vi "FT10_Fornax Send MonopolarCommand.vi"(8 "error in":errorcluster, 10 "Set Monopolar Command Cluster in":T12={"Serial Number"="CAMM_INTERNAL_GENERIC", "EnergyChannelID"=enum."EC_MONO_1", "CutMode"=enum."SPRAY_MODE", "CoagMode"=enum."SPRAY_MODE", "CutPowerCommand"=enum."POWER_NO_CHANGE", "CoagPowerCommand"=enum."POWER_NO_CHANGE", "Fornax Set Monopolar Command"=FALSE}, 11 "Message Handling Cluster in":T1={"Fornax Connected?"=refnum, "Unitherm Connected?"=refnum, "M4X Connected?"=refnum, "Unitherm Connect/Disconnect"=refnum, "Fornax Connection"=refnum, "UNITHERM Connection"="", "M4X Connection"=0, "PXI-7854R FPGA Reference"=refnum, "PXI-7854R Connected?"=refnum, "Fornax Connect/Disconnect"=refnum, "7854 Connect/Disconnect"=refnum, "M4X Connect/Disconnect"=refnum, "Config Cluster"={"Unitherm Port"="COM4", "Simulate Values"=TRUE}, "Log Queue"=refnum, "Log Analysis Cluster"={"RMS"=0.0, "Envelope Frequency"=0.0, "Peak"=0.0, "Crest Factor"=0.0, "Duty Cyle %"=0.0, "P-P"=0.0, "Frequency"=0.0, "THD"=0.0, "Postive Peak"=0.0, "Negative Peak"=0.0, "Mag_H1"=0.0, "Phase_H1"=0.0, "Mag_H3"=0.0, "Phase_H3"=0.0, "Mag_H5"=0.0, "Phase_H5"=0.0}, "Log Waveform Cluster"={"t0"=timestamp(0 s since 1904-01-01), "dt"=1.0, "Y"=[]}, "Log Time"=timestamp(0 s since 1904-01-01), "Log Flag"=FALSE}) -> (0 "error out":errorcluster, 2 "Set Monopolar Command Cluster out":T12={"Serial Number"="CAMM_INTERNAL_GENERIC", "EnergyChannelID"=enum."EC_MONO_1", "CutMode"=enum."SPRAY_MODE", "CoagMode"=enum."SPRAY_MODE", "CutPowerCommand"=enum."POWER_NO_CHANGE", "CoagPowerCommand"=enum."POWER_NO_CHANGE", "Fornax Set Monopolar Command"=FALSE}, 3 "Message Handling Cluster out":T1={"Fornax Connected?"=refnum, "Unitherm Connected?"=refnum, "M4X Connected?"=refnum, "Unitherm Connect/Disconnect"=refnum, "Fornax Connection"=refnum, "UNITHERM Connection"="", "M4X Connection"=0, "PXI-7854R FPGA Reference"=refnum, "PXI-7854R Connected?"=refnum, "Fornax Connect/Disconnect"=refnum, "7854 Connect/Disconnect"=refnum, "M4X Connect/Disconnect"=refnum, "Config Cluster"={"Unitherm Port"="COM4", "Simulate Values"=TRUE}, "Log Queue"=refnum, "Log Analysis Cluster"={"RMS"=0.0, "Envelope Frequency"=0.0, "Peak"=0.0, "Crest Factor"=0.0, "Duty Cyle %"=0.0, "P-P"=0.0, "Frequency"=0.0, "THD"=0.0, "Postive Peak"=0.0, "Negative Peak"=0.0, "Mag_H1"=0.0, "Phase_H1"=0.0, "Mag_H3"=0.0, "Phase_H3"=0.0, "Mag_H5"=0.0, "Phase_H5"=0.0}, "Log Waveform Cluster"={"t0"=timestamp(0 s since 1904-01-01), "dt"=1.0, "Y"=[]}, "Log Time"=timestamp(0 s since 1904-01-01), "Log Flag"=FALSE})   [LabVIEW 2015]
uses:
  Controls/Control_Fornax Set Monopolar Command Cluster.ctl
  Controls/Control_Fornax Set Monopolar Command - Serial Number String.ctl
  Controls/Control_Fornax Set Monopolar Command - Energy Channel ID Enum.ctl
  Controls/Control_Fornax Set Monopolar Command - Cut Mode Enum.ctl
  Controls/Control_Fornax Set Monopolar Command - Coag Mode Enum.ctl
  Controls/Control_Fornax Set Monopolar Command - Cut Power Command Enum.ctl
  Controls/Control_Fornax Set Monopolar Command - Coag Power Command Enum.ctl
  Controls/Control_Fornax Set Monopolar Command Bool.ctl
  Controls/Control_Message Handling Cluster.ctl
  Controls/Control_M4X Connection.ctl
  Controls/Control_PXI-7854R FPGA Reference.ctl
  Controls/Control_Config Cluster.ctl
  Controls/Control_Config Unitherm Port.ctl
  Controls/Control_Config Simulate Values.ctl
  Controls/Control_Log Queue.ctl
  Controls/Control_Log Cluster.ctl
  Controls/Control_Log Time.ctl
  Controls/Control_Log Waveform Cluster.ctl
  Controls/Control_Log Analysis Cluster.ctl
  Controls/Control_Log Flag.ctl
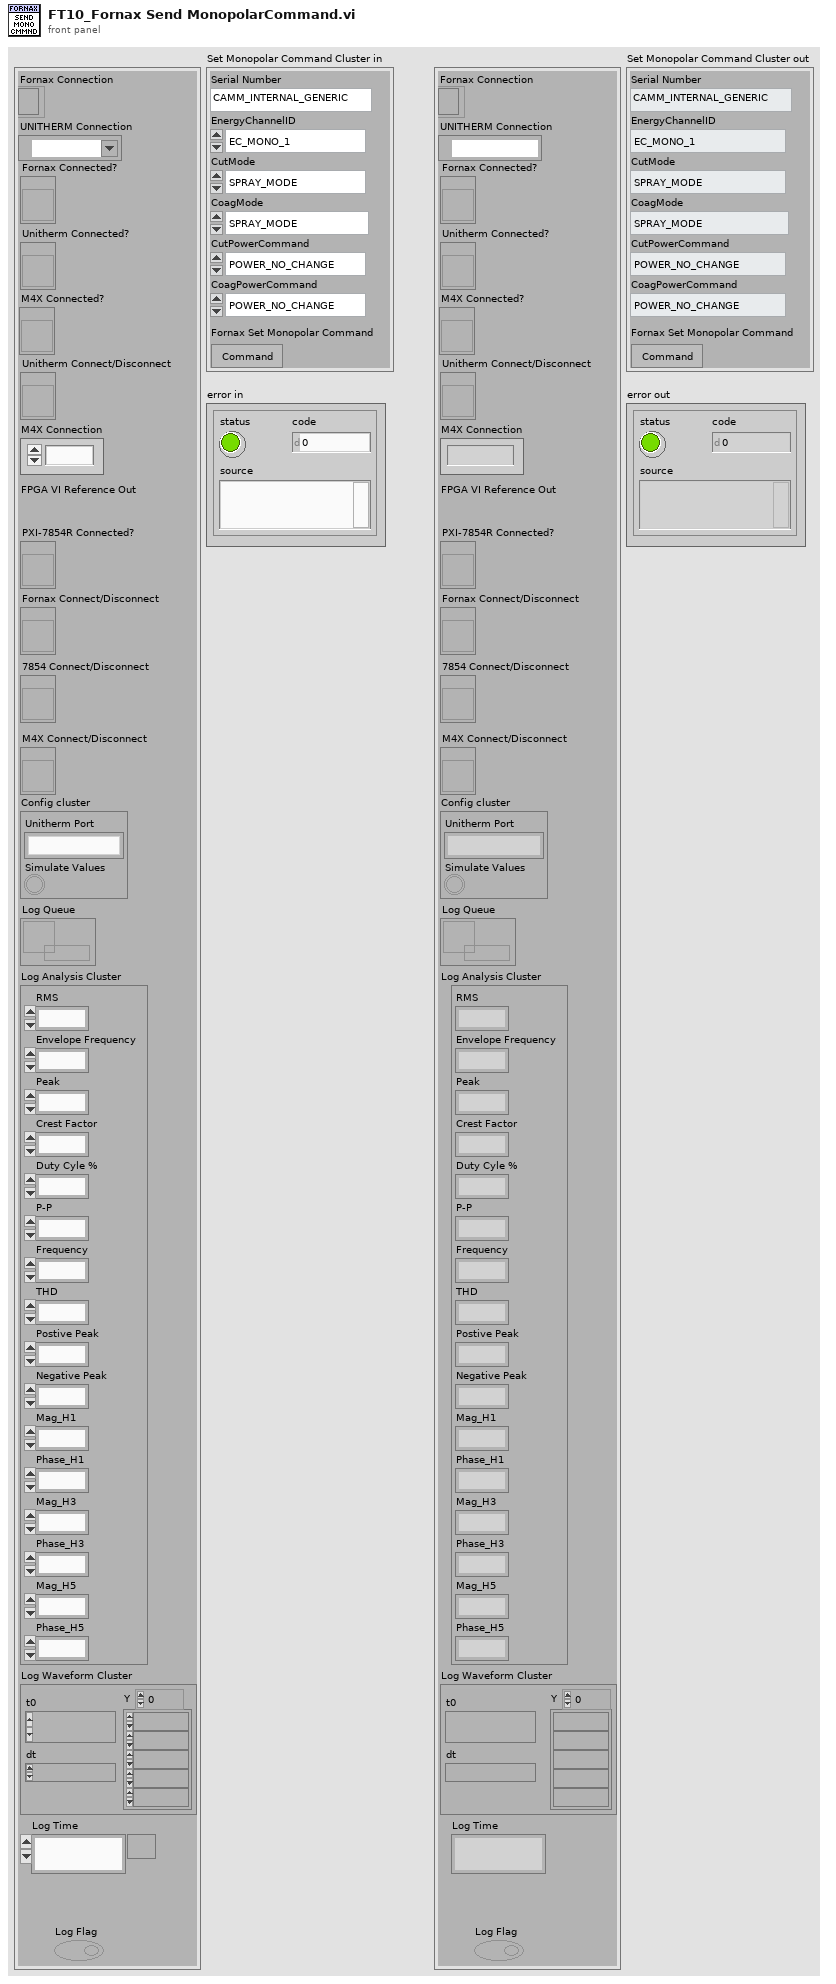
[diagram p1: front panel]
types:
  T1 = typedef "Control_Message Handling Cluster.ctl" = cluster{"Fornax Connected?":refnum<vi>, "Unitherm Connected?":refnum<vi>, "M4X Connected?":refnum<vi>, "Unitherm Connect/Disconnect":refnum<vi>, "Fornax Connection":refnum<k5>, "UNITHERM Connection":refnum<visa-resource-name>, "M4X Connection":T2, "PXI-7854R FPGA Reference":T3, "PXI-7854R Connected?":refnum<vi>, "Fornax Connect/Disconnect":refnum<vi>, "7854 Connect/Disconnect":refnum<vi>, "M4X Connect/Disconnect":refnum<vi>, "Config Cluster":T4, "Log Queue":T7, "Log Analysis Cluster":T8, "Log Waveform Cluster":T9, "Log Time":T10, "Log Flag":T11}
  T2 = typedef "Control_M4X Connection.ctl" = u32
  T3 = typedef "Control_PXI-7854R FPGA Reference.ctl" = refnum<k20>
  T4 = typedef "Control_Config Cluster.ctl" = cluster{"Unitherm Port":T5, "Simulate Values":T6}
  T5 = typedef "Control_Config Unitherm Port.ctl" = string
  T6 = typedef "Control_Config Simulate Values.ctl" = bool
  T7 = typedef "Control_Log Queue.ctl" = refnum<queue>
  T8 = typedef "Control_Log Analysis Cluster.ctl" = cluster{"RMS":dbl, "Envelope Frequency":dbl, "Peak":dbl, "Crest Factor":dbl, "Duty Cyle %":dbl, "P-P":dbl, "Frequency":dbl, "THD":dbl, "Postive Peak":dbl, "Negative Peak":dbl, "Mag_H1":dbl, "Phase_H1":dbl, "Mag_H3":dbl, "Phase_H3":dbl, "Mag_H5":dbl, "Phase_H5":dbl}
  T9 = typedef "Control_Log Waveform Cluster.ctl" = waveform(dbl)
  T10 = typedef "Control_Log Time.ctl" = timestamp
  T11 = typedef "Control_Log Flag.ctl" = bool
  T12 = typedef "Control_Fornax Set Monopolar Command Cluster.ctl" = cluster{"Serial Number":T13, "EnergyChannelID":T14, "CutMode":T15, "CoagMode":T16, "CutPowerCommand":T17, "CoagPowerCommand":T18, "Fornax Set Monopolar Command":T19}
  T13 = typedef "Control_Fornax Set Monopolar Command - Serial Number String.ctl" = string
  T14 = typedef "Control_Fornax Set Monopolar Command - Energy Channel ID Enum.ctl" = enum16{"EC_MONO_1", "EC_BIPOLAR", "EC_MONO_2", "EC_ADVANCED", "NUM_ENERGY_CHANNELS", "EC_NOT_USED"}
  T15 = typedef "Control_Fornax Set Monopolar Command - Cut Mode Enum.ctl" = enum16{"SPRAY_MODE", "CUT_MODE", "BLEND_MODE", "FULGERATE_MODE", "BIPOLAR_MODE", "VESSEL_SEALING_MODE", "VALLEYLAB_MODE", "BIPOLAR_RESECTION_CUT_MODE", "BIPOLAR_RESECTION_COAG_MODE", "AUTOBIPOLAR_MODE", "VIPER_HLA", "SOFT_COAG_MODE", "NUM_ENERGY_MODES"}
  T16 = typedef "Control_Fornax Set Monopolar Command - Coag Mode Enum.ctl" = enum16{"SPRAY_MODE", "CUT_MODE", "BLEND_MODE", "FULGERATE_MODE", "BEPOLAR_MODE", "VESSEL_SEALING_MODE", "VALLEYLAB_MODE", "BIPOLAR_RESECTION_CUT_MODE", "BIPOLAR_RESECTION_COAG_MODE", "AUTOBIPOLAR_MODE", "VIPER_HLA", "SOFT_COAG_MODE", "NUM_ENERGY_MODES"}
  T17 = typedef "Control_Fornax Set Monopolar Command - Cut Power Command Enum.ctl" = enum16{"POWER_NO_CHANGE", "POWER_INCREASE", "POWER_DECREASE", "POWER_INCREASE_REPEAT", "POWER_DECREASE_REPEAT"}
  T18 = typedef "Control_Fornax Set Monopolar Command - Coag Power Command Enum.ctl" = enum16{"POWER_NO_CHANGE", "POWER_INCREASE", "POWER_DECREASE", "POWER_INCREASE_REPEAT", "POWER_DECREASE_REPEAT"}
  T19 = typedef "Control_Fornax Set Monopolar Command Bool.ctl" = bool
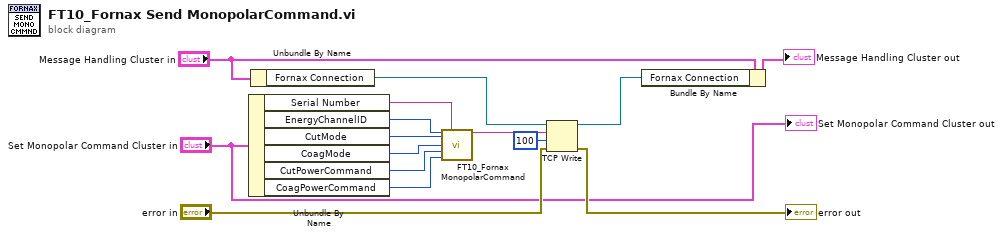
[diagram p0: block diagram]
diagram:
  n1 = Unbundle By Name("Set Monopolar Command Cluster in") -> ("Serial Number"=w14:T13, "EnergyChannelID"=w13:T14, "CutMode"=w12:T15, "CoagMode"=w9:T16, "CutPowerCommand"=w10:T17, "CoagPowerCommand"=w11:T18)
  n2 = Unbundle By Name("Message Handling Cluster in") -> ("Fornax Connection"=w3:refnum<k5>)
  n3 = call "FT10_Fornax MonopolarCommand.vi"("EnergyChannelID"=w13, "Serial Number"=w14, "CutMode"=w12, "CoagMode"=w9, "CutPowerCommand"=w10, "CoagPowerCommand"=w11) -> ("JSON Command"=w8:string)  [unwired: 9 in]
  n4 = TCP Write(connection ID=w3, data in=w8, error in (no error)="error in", 9:100 ("timeout ms (25000)")) -> (connection ID out=w1:refnum<k5>, error out=→"error out":errorcluster)  [unwired: 1 out]
  n5 = Bundle By Name(cluster="Message Handling Cluster in", "Fornax Connection"=w1) -> (→"Message Handling Cluster out":T1)
  "Set Monopolar Command Cluster out" <- "Set Monopolar Command Cluster in"
